vi "Fetch Waveform.vi"(8 "error in (no error)":errorcluster, 11 "NI DMM in":refnum<class "NI DMM.lvclass">) -> (0 "error out":errorcluster, 2 "Data":variant, 3 "NI DMM out":refnum<class "NI DMM.lvclass">)   [LabVIEW 2020, in "NI DMM.lvlib" / "NI DMM.lvclass"]
uses:
  NI DMM.lvclass
  NI DMM.lvclass/NI DMM.ctl
  <instrlib>/niDMM/nidmm.llb/niDMM Fetch Waveform (floating point array).vi
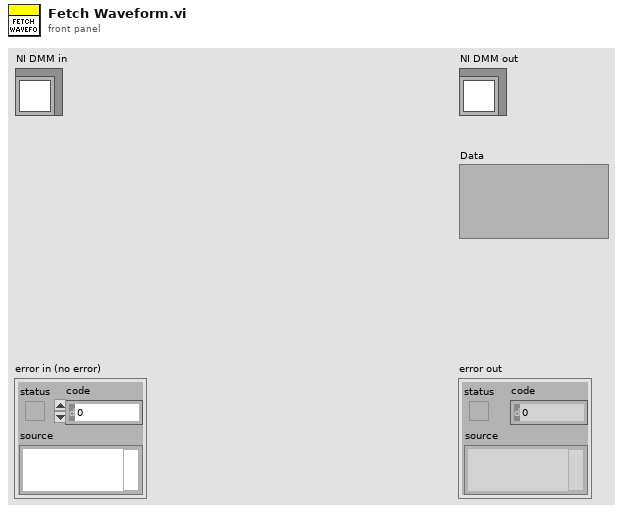
[diagram p1: front panel]
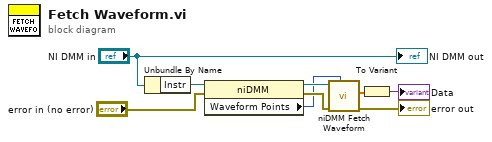
[diagram p0: block diagram]
diagram:
  n1 = Unbundle By Name("NI DMM in") -> ("Instr"=w8:refnum<k15>)
  n2 = property class="niDMM"(reference=w8, error in="error in (no error)") -> (reference out=w7:refnum<k15>, error out=w3:errorcluster, "Waveform Points"=w1:i32)
  n3 = call-poly <instrlib>:"niDMM Fetch Waveform.vi"("Number To Fetch"=w1, "error in (no error)"=w3, "instrument handle"=w7) -> ("error out"=→"error out":errorcluster, "Measurements"=w6:dbl[])  [unwired: 5 in, 2 out]
  n4 = To Variant(anything=w6) -> (Variant=→"Data":variant)
  "NI DMM out" <- "NI DMM in"
